vi "Configure Instrument.vi"(8 "error in (no error)":errorcluster, 11 "Instrument.Lockin":refnum<class "Instrument.Lockin.lvclass">) -> (0 "error out":errorcluster, 3 "Instrument.Lockin out":refnum<class "Instrument.Lockin.lvclass">)   [LabVIEW 2016, in "Instrument.Lockin.lvclass"]
uses:
  Instrument.Lockin.lvclass
  Instrument.Lockin.lvclass/Instrument.Lockin.ctl
  <userlib>/LevyLab/Levylab Instruments/SMOs/Instrument/Instrument.lvclass
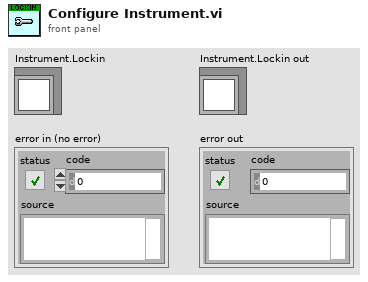
[diagram p1: front panel]
types:
  T1 = typedef "Instrument.Lockin.lvclass/Instrument.Lockin.Configuration--Cluster.ctl" = cluster{"Channels: AO":T2, "Channels: REF":T9, "REF Filter":cluster{"LP cutoff (Hz)":dbl, "LP prefilter":bool, "60 Hz prefilter":bool, "REF filter":T12}, "Amplifers":cluster{"offsets":dbl[], "Gain":dbl[], "Amplifiers":T13}, "DAQ":cluster{"sampling":T14, "sample mode":i32, "buffer size (S)":u32}, "Calibration":cluster{"Cal Info":T15[]}, "AI Configuration":T16, "AO Configuration":T21}
  T2 = typedef "LockinDAQ.lvclass/AO-cluster.ctl" = cluster{"AO Amp (V)":T3, "AO DC (V)":T4, "AO f (Hz)":T5, "AO Phase (°)":T6, "Function":T7, "I+":bool[], "Sweeping":bool[]}
  T3 = typedef "LockinDAQ.lvclass/AO_Amp-array.ctl" = dbl[]
  T4 = typedef "LockinDAQ.lvclass/AO_DC-array.ctl" = dbl[]
  T5 = typedef "LockinDAQ.lvclass/AO_f-array.ctl" = dbl[]
  T6 = typedef "LockinDAQ.lvclass/AO_phi-array.ctl" = dbl[]
  T7 = typedef "LockinDAQ.lvclass/Function-array.ctl" = T8[]
  T8 = typedef "LockinDAQ.lvclass/Function-enum.ctl" = enum16{"Sine", "Triangle", "Square", "Sawtooth"}
  T9 = typedef "LockinDAQ.lvclass/REF-cluster.ctl" = cluster{"REF f (Hz)":T10, "REF phi (°)":T11}
  T10 = typedef "LockinDAQ.lvclass/REF_f-array.ctl" = dbl[]
  T11 = typedef "LockinDAQ.lvclass/REF_phi-array.ctl" = dbl[]
  T12 = typedef "LockinDAQ.lvclass/REF filter-cluster.ctl" = cluster{"TC (s)":dbl, "order":i32}
  T13 = typedef "LockinDAQ.lvclass/AmplifierType-enum.ctl" = enum16{"Manual", "Krohn Hite", "Femto"}
  T14 = typedef "LockinDAQ.lvclass/Sampling.ctl" = cluster{"Fs":dbl, "#s":i32}
  T15 = typedef "LockinDAQ.lvclass/Cal Info - Cluster.ctl" = cluster{"Active Device":tag, "SelfCal.LastDate/Time":timestamp, "SelfCal.LastTemp":dbl, "DevTemp":dbl, "calibration due?":bool}
  T16 = typedef "LockinDAQ.lvclass/AI.config-array.ctl" = T17[]
  T17 = typedef "LockinDAQ.lvclass/AI.config-cluster.ctl" = cluster{"AI.channels":tag, "AI.Coupling":T18, "AI.Range":T19, "input terminal configuration":i32, "DAQ Type":T20}
  T18 = typedef "LockinDAQ.lvclass/AI.coupling-enum.ctl" = u16
  T19 = typedef "LockinDAQ.lvclass/446xAI-enum.ctl" = enum16{"±0.316 V", "±1.00 V", "±3.16 V", "±10.0 V", "±31.6 V", "±42.4 V"}
  T20 = typedef "LockinDAQ.lvclass/DAQType-enum.ctl" = enum16{"None", "USB 4431", "PXI 446x"}
  T21 = typedef "LockinDAQ.lvclass/AO.config-array.ctl" = T22[]
  T22 = typedef "LockinDAQ.lvclass/AO.config-cluster.ctl" = cluster{"AO.channels":tag, "AO.Range":T23, "output terminal configuration":i32, "DAQ Type":T20}
  T23 = typedef "LockinDAQ.lvclass/446xAO-enum.ctl" = enum16{"±0.1 V", "±1.0 V", "±10.0 V"}
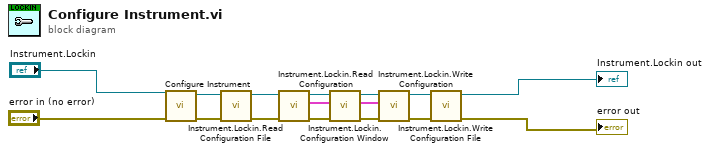
[diagram p0: block diagram]
diagram:
  n1 = call-parent "Configure Instrument.vi"("error in (no error)"="error in (no error)", "Instrument in"="Instrument.Lockin") -> ("error out"=w11:errorcluster, "Instrument out"=w13:refnum<class "Instrument.Lockin.lvclass">)  [unwired: 8 in]
  n2 = call "Instrument.Lockin.Read Configuration File.vi"("error in (no error)"=w11, "Instrument.Lockin"=w13) -> ("error out"=w10:errorcluster, "Instrument.Lockin out"=w9:refnum<class "Instrument.Lockin.lvclass">)  [unwired: 8 in]
  n3 = call "Instrument.Lockin.Read Configuration.vi"("error in (no error)"=w10, "Instrument.Lockin"=w9) -> ("error out"=w7:errorcluster, "Configuration"=w2:T1, "Instrument.Lockin out"=w8:refnum<class "Instrument.Lockin.lvclass">)  [unwired: 7 in]
  n4 = call "Instrument.Lockin.Configuration Window.vi"("error in (no error)"=w7, "Ex Configuration"=w2, "Instrument.Lockin"=w8) -> ("error out"=w6:errorcluster, "output cluster"=w1:T1, "Instrument.Lockin out"=w5:refnum<class "Instrument.Lockin.lvclass">)  [unwired: 6 in]
  n5 = call "Instrument.Lockin.Write Configuration.vi"("error in (no error)"=w6, "Configuration"=w1, "Instrument.Lockin"=w5) -> ("error out"=w3:errorcluster, "Instrument.Lockin out"=w4:refnum<class "Instrument.Lockin.lvclass">)  [unwired: 7 in]
  n6 = call "Instrument.Lockin.Write Configuration File.vi"("error in (no error)"=w3, "Instrument.Lockin"=w4) -> ("error out"=→"error out":errorcluster, "Instrument.Lockin out"=→"Instrument.Lockin out":refnum<class "Instrument.Lockin.lvclass">)  [unwired: 8 in]
